vi "HypoToDistInches.vi"(1 "Hypotenuse (ft)":dbl) -> (0 "Distance":dbl)   [LabVIEW 2015]
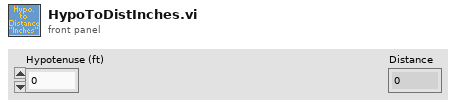
[diagram p1: front panel]
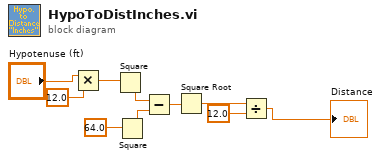
[diagram p0: block diagram]
diagram:
  n1 = Multiply(x="Hypotenuse (ft)", y=12.0) -> (x*y=w6:dbl)
  n2 = Square(x=w6) -> (x^2=w8:dbl)
  n3 = Square(x=64.0) -> (x^2=w7:dbl)
  n4 = Subtract(x=w8, y=w7) -> (x-y=w10:dbl)
  n5 = Square Root(x=w10) -> (sqrt(x)=w2:dbl)
  n6 = Divide(x=w2, y=12.0) -> (x/y=→"Distance":dbl)
